vi "astrom_test.vi"() -> ()   [LabVIEW 2010]
panel:
  out "ImgRA [°]":dbl format="%.6f"
  out "ImgDEC [°]":dbl format="%.5f"
  in  "settablexy":bool
  in  "setpixel":bool
  in  "Image Y":dbl
  in  "Image X":dbl
  in  "RA":dbl format="%<%H:%M:%S%2u>t"
  in  "DEC":dbl format="%<%H:%M:%S%1u>t"
  out "ZoomIN":sgl[][](graph)
  in  "Table Y":dbl format="%.2f"
  in  "Table X":dbl format="%.2f"
  in  "setradec":bool
  in  "readcursor":bool
  out "Imgage Data":sgl[][](array[numeric])
  out "ImgRA [sec]":dbl format="%<%H:%M:%S%2u>t"
  out "ImgDEC [sec]":dbl format="%<%H:%M:%S%1u>t"
  in  "Plot Size [arcmin]":dbl
  in  "redraw":bool
  in  "extast":bool
  in  "quit":bool
  in  "DEC(DD:MM:SS)":dbl format="%<%H:%M:%S>t"
  in  "RA (HH:MM:SS.S)":dbl format="%<%H:%M:%S%1u>t"
  out "Field Astrometry":T1
  out "Table Astrometry":T1
  out "Image Astrometry":T1
  in  "Ref y (pas)":dbl
  in  "Ref x (pas)":dbl
  in  "effective rotation (°)":dbl step=5.0
  in  "scale (\"/pas)":dbl
  out "XY Graph":cluster{dbl[], dbl[]}[](graph)
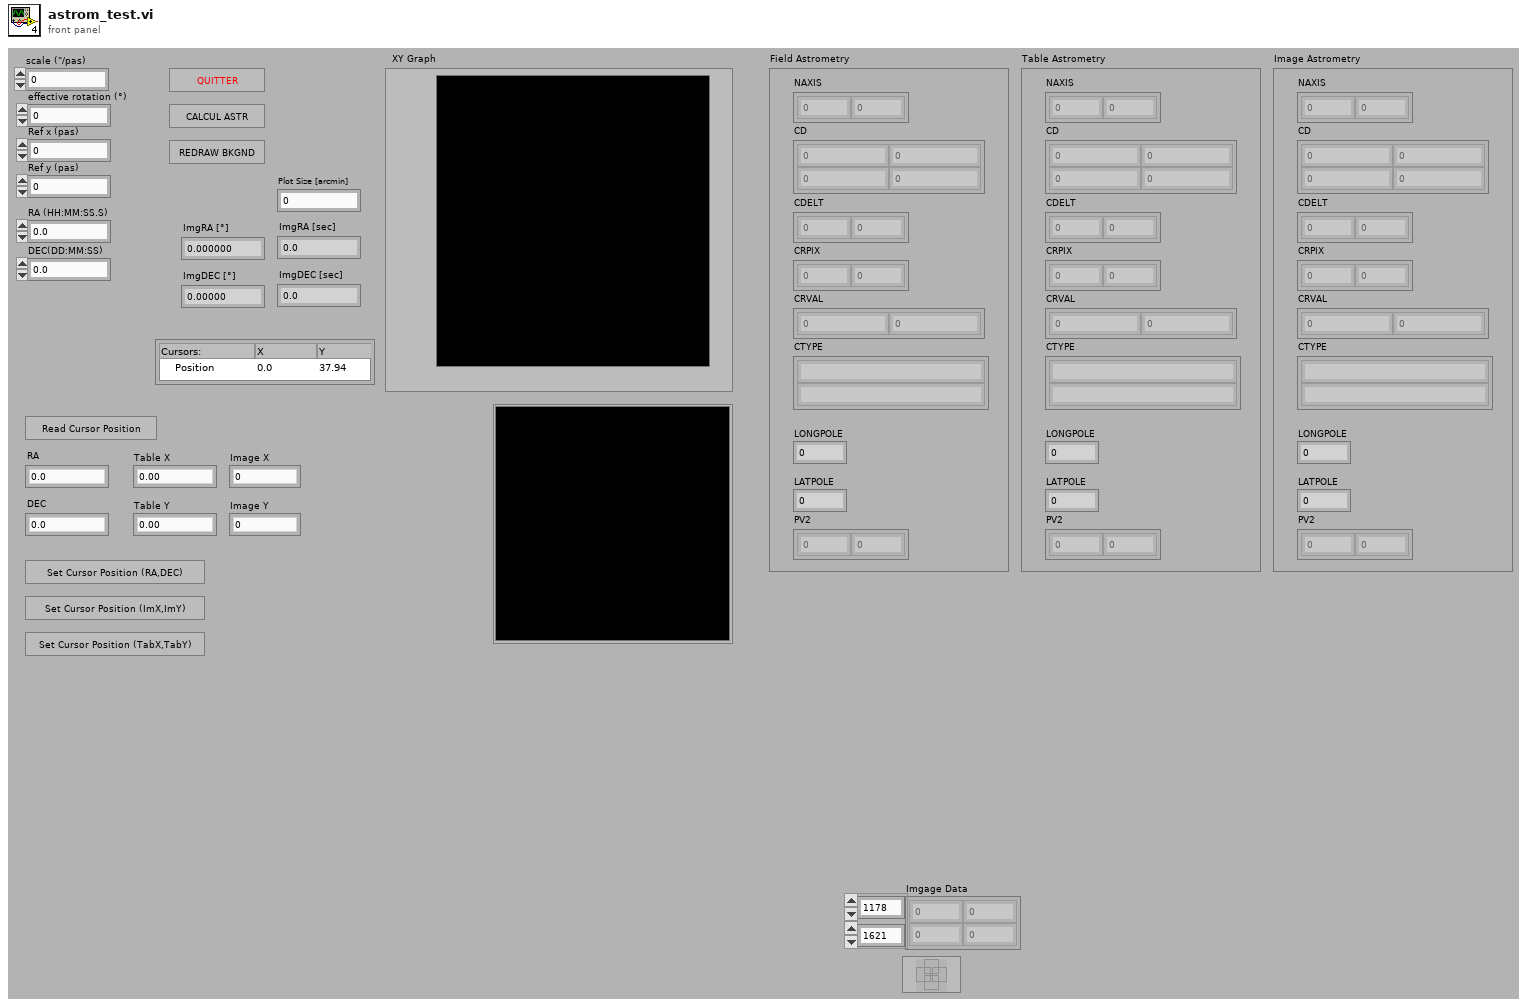
[diagram p1: front panel]
types:
  T1 = cluster{"NAXIS":dbl[], "CD":dbl[][], "CDELT":dbl[], "CRPIX":dbl[], "CTYPE":string[], "CRVAL":dbl[], "LONGPOLE":dbl, "LATPOLE":dbl, "PV2":dbl[]}
  T2 = typedef "LVRangeTypeDef.ctl" = cluster{"Minimum":dbl, "Maximum":dbl, "Increment":dbl, "Minor Increment":dbl, "Start":dbl}
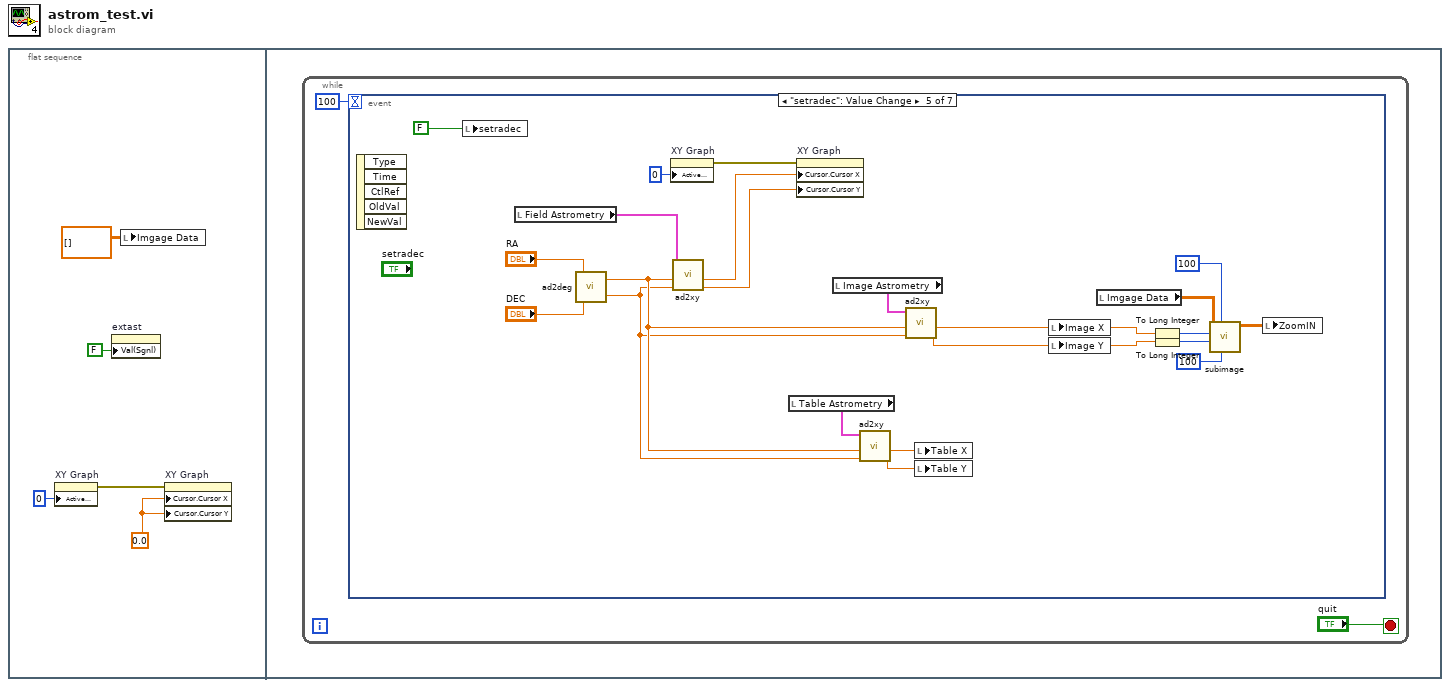
[diagram p0: block diagram]
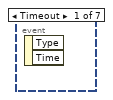
[diagram p2: hidden frame]
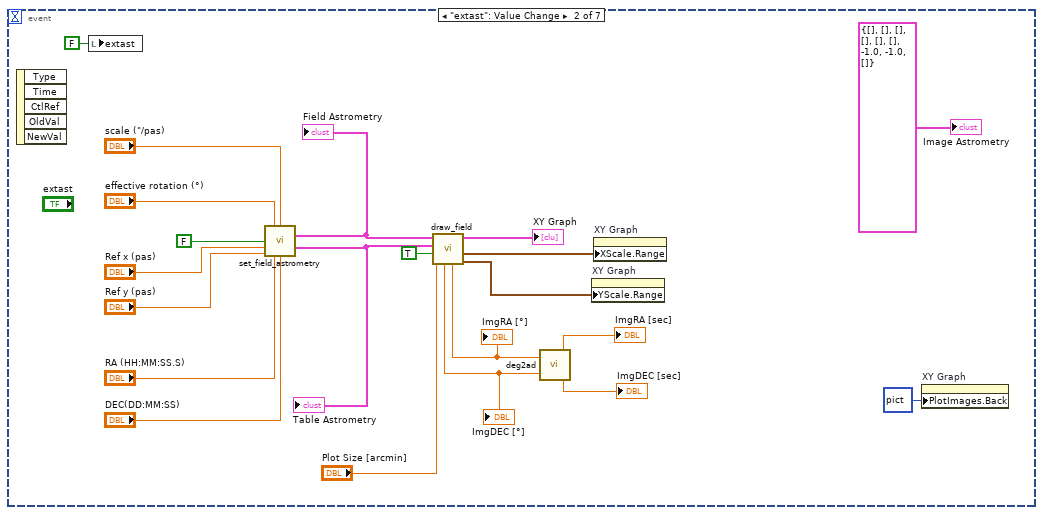
[diagram p3: hidden frame]
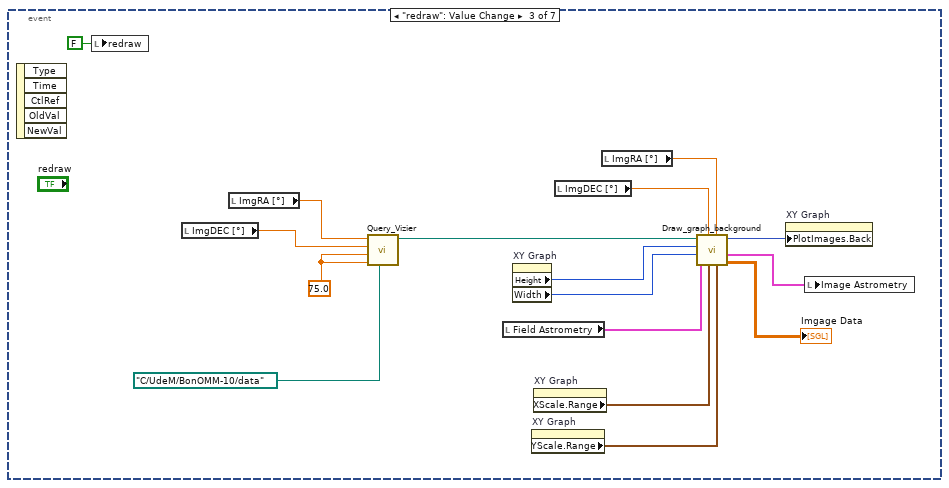
[diagram p4: hidden frame]
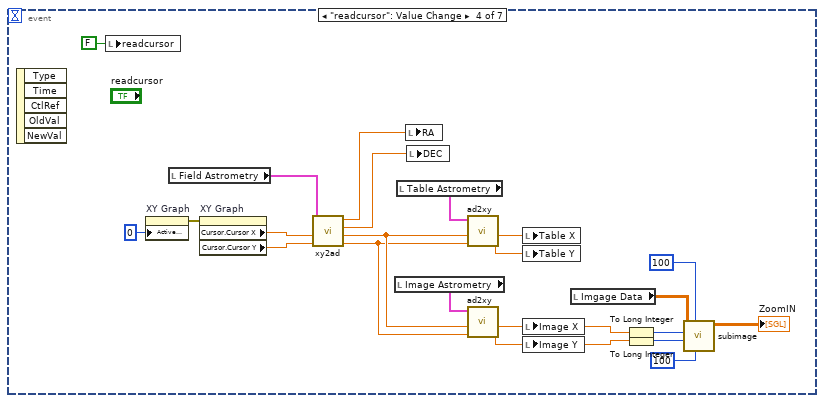
[diagram p5: hidden frame]
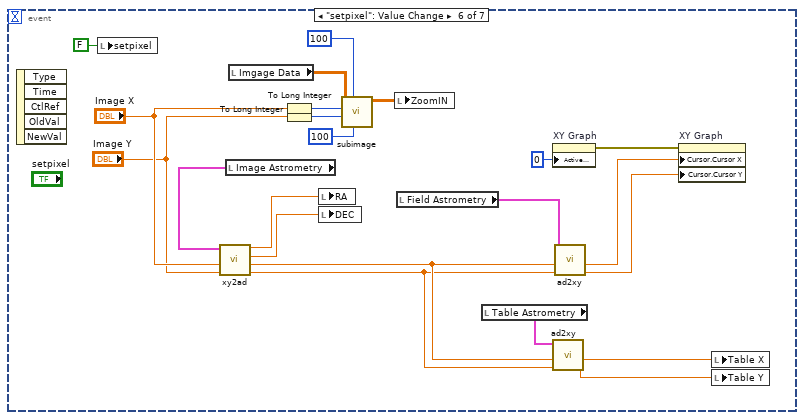
[diagram p6: hidden frame]
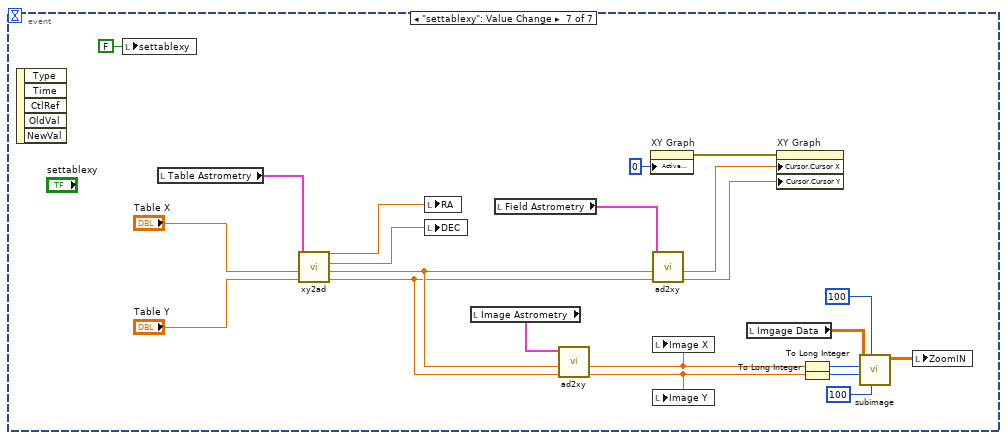
[diagram p7: hidden frame]
diagram:
  n1 = flat-sequence {
    frame #0 {
      w1 = 0.0
      n2 = property on="XY Graph" class="XYGraph (strict)"("Active Cursor"=u32 0) -> (error out=w2:errorcluster)  [unwired: 2 in, 1 out]
      n3 = property on="extast" class="Bool (strict)"("Val(Sgnl)"=FALSE ("Value (Signaling)")) -> ()  [unwired: 2 in, 2 out]
      n4 = local write "Imgage Data"(sgl[][] [] ("Imgage Data")) -> ()
      n5 = property on="XY Graph" class="XYGraph (strict)"(error in=w2, "Cursor.Cursor X"=w1, "Cursor.Cursor Y"=w1) -> ()  [unwired: 1 in, 2 out]
    }
    frame #1 {
      n6 = while {
        stop <- "quit" stop-if-true
        n7 = event shown="[4] \"setradec\": Value Change" {
          selector: _ -> [_ _ _ _ _ _ _]
          dyn-events: _ -> [_ _ _ _ _ _ _]
          timeout: 100 -> [_ _ _ _ _ _ _]
          event Timeout {
            n8 = event-data() -> ()  [unwired: 1 in, 2 out]
          }
          event "extast": Value Change {
            n9 = event-data() -> ()  [unwired: 1 in, 5 out]
            n10 = local write "extast"(FALSE ("extast")) -> ()
            n11 = call "set_field_astrometry.vi"("effective rotation (°)"="effective rotation (°)", "scale (\"/pas)"="scale (\"/pas)", "Use Center?"=FALSE, "Ref x (pas)"="Ref x (pas)", "Ref y (pas)"="Ref y (pas)", "RA (HH:MM:SS.S)"="RA (HH:MM:SS.S)", "DEC(DD:MM:SS)"="DEC(DD:MM:SS)") -> ("Field Astrometry"=w21:T1, "Table Astrometry"=w22:T1)  [unwired: 7 in]
            "Table Astrometry" <- w22
            "Field Astrometry" <- w21
            n12 = call "draw_field.vi"("margin/size"="Plot Size [arcmin]", "Ues Constant Size ?"=TRUE, "Table_Astrometry"=w22, "Field_Astrometry"=w21) -> ("Y Scale.Range"=w15:T2, "X Scale.Range"=w16:T2, "TableXYPos"=→"XY Graph":cluster{dbl[], dbl[]}[], "ImgRA"=w11:dbl, "ImgDEC"=w10:dbl)  [unwired: 3 in]
            "ImgRA [°]" <- w11
            "ImgDEC [°]" <- w10
            n13 = call "deg2ad.vi"("DEC (°)"=w10, "RA (°)"=w11) -> ("DEC (sec)"=→"ImgDEC [sec]":dbl, "RA (sec)"=→"ImgRA [sec]":dbl)
            n14 = property on="XY Graph" class="XYGraph (strict)"("YScale.Range"=w15) -> ()  [unwired: 2 in, 2 out]
            n15 = property on="XY Graph" class="XYGraph (strict)"("XScale.Range"=w16) -> ()  [unwired: 2 in, 2 out]
            n16 = property on="XY Graph" class="XYGraph (strict)"("PlotImages.Back"=picture data[5B] ("Plot Images:Back")) -> ()  [unwired: 2 in, 2 out]
            "Image Astrometry" <- T1 {"NAXIS"=[], "CD"=[], "CDELT"=[], "CRPIX"=[], "CTYPE"=[], "CRVAL"=[], "LONGPOLE"=-1.0, "LATPOLE"=-1.0, "PV2"=[]} ("Image Astrometry")
          }
          event "redraw": Value Change {
            w31 = 75.0 ("Height")
            n17 = event-data() -> ()  [unwired: 1 in, 5 out]
            n18 = local write "redraw"(FALSE ("redraw")) -> ()
            n19 = local read "ImgDEC [°]"() -> (w32:dbl)
            n20 = local read "ImgRA [°]"() -> (w33:dbl)
            n21 = call "Query_Vizier.vi"("Folder"=path "C:/UdeM/BonOMM-10/data", "Width"=w31, "Height"=w31, "DEC"=w32, "RA"=w33) -> ("Path2Image"=w29:path)  [unwired: 5 in, 1 out]
            n22 = local read "Field Astrometry"() -> (w40:T1)
            n23 = property on="XY Graph" class="XYGraph (strict)"() -> ("Height"=w42:u32, "Width"=w41:u32)  [unwired: 2 in, 2 out]
            n24 = property on="XY Graph" class="XYGraph (strict)"() -> ("YScale.Range"=w38:T2)  [unwired: 2 in, 2 out]
            n25 = property on="XY Graph" class="XYGraph (strict)"() -> ("XScale.Range"=w39:T2)  [unwired: 2 in, 2 out]
            n26 = local read "ImgDEC [°]"() -> (w36:dbl)
            n27 = local read "ImgRA [°]"() -> (w37:dbl)
            n28 = call "Draw_graph_background.vi"("Y Scale.Range"=w38, "ImgRA"=w37, "X Scale.Range"=w39, "ImgDEC"=w36, "Field Astrometry"=w40, "New Width"=w41, "New Height"=w42, "path"=w29) -> ("ImgData"=→"Imgage Data":sgl[][], "Astrometry"=w35:T1, "Images"=w43:picture)  [unwired: 1 in]
            n29 = property on="XY Graph" class="XYGraph (strict)"("PlotImages.Back"=w43) -> ()  [unwired: 2 in, 2 out]
            n30 = local write "Image Astrometry"(w35) -> ()
          }
          event "readcursor": Value Change {
            n31 = event-data() -> ()  [unwired: 1 in, 5 out]
            n32 = local write "readcursor"(FALSE ("readcursor")) -> ()
            n33 = property on="XY Graph" class="XYGraph (strict)"("Active Cursor"=u32 0) -> (error out=w65:errorcluster)  [unwired: 2 in, 1 out]
            n34 = local read "Field Astrometry"() -> (w62:T1)
            n35 = property on="XY Graph" class="XYGraph (strict)"(error in=w65) -> ("Cursor.Cursor X"=w64:dbl, "Cursor.Cursor Y"=w63:dbl)  [unwired: 1 in, 2 out]
            n36 = call "xy2ad.vi"("Y (px)"=w63, "X (px)"=w64, "Astrometry"=w62) -> ("DEC (°)"=w59:dbl, "RA (°)"=w60:dbl, "DEC (HH:MM:SS)"=w56:dbl, "RA (HH:MM:SS.S)"=w57:dbl)  [unwired: 5 in]
            n37 = local read "Image Astrometry"() -> (w58:T1)
            n38 = local read "Table Astrometry"() -> (w61:T1)
            n39 = local write "RA"(w57) -> ()
            n40 = local write "DEC"(w56) -> ()
            n41 = call "ad2xy.vi"("DEC"=w59, "RA"=w60, "Astrometry"=w61) -> ("Y"=w54:dbl, "X"=w55:dbl)  [unwired: 6 in, 1 out]
            n42 = call "ad2xy.vi"("DEC"=w59, "RA"=w60, "Astrometry"=w58) -> ("Y"=w50:dbl, "X"=w51:dbl)  [unwired: 6 in, 1 out]
            n43 = local write "Table X"(w55) -> ()
            n44 = local write "Table Y"(w54) -> ()
            n45 = local write "Image X"(w51) -> ()
            n46 = local write "Image Y"(w50) -> ()
            n47 = local read "Imgage Data"() -> (w47:sgl[][])
            n48 = To Long Integer(number=w51) -> (32bit integer=w53:i32)
            n49 = To Long Integer(number=w50) -> (32bit integer=w52:i32)
            n50 = call "subimage.vi"("Ysz/2"=100, "Xsz/2"=100, "Yc"=w52, "Xc"=w53, "ImgData"=w47) -> ("SubImg"=→"ZoomIN":sgl[][])  [unwired: 6 in]
          }
          event "setradec": Value Change {
            n51 = event-data() -> ()  [unwired: 1 in, 5 out]
            n52 = local write "setradec"(FALSE ("setcursor")) -> ()
            n53 = local read "Field Astrometry"() -> (w87:T1)
            n54 = call "ad2deg.vi"("DEC (sec)"="DEC", "RA (sec)"="RA") -> ("DEC (°)"=w67:dbl, "RA (°)"=w68:dbl)
            n55 = property on="XY Graph" class="XYGraph (strict)"("Active Cursor"=u32 0) -> (error out=w86:errorcluster)  [unwired: 2 in, 1 out]
            n56 = call "ad2xy.vi"("DEC"=w67, "RA"=w68, "Astrometry"=w87) -> ("Y"=w84:dbl, "X"=w85:dbl)  [unwired: 6 in, 1 out]
            n57 = local read "Table Astrometry"() -> (w74:T1)
            n58 = property on="XY Graph" class="XYGraph (strict)"(error in=w86, "Cursor.Cursor X"=w85, "Cursor.Cursor Y"=w84) -> ()  [unwired: 1 in, 2 out]
            n59 = local read "Image Astrometry"() -> (w82:T1)
            n60 = call "ad2xy.vi"("DEC"=w67, "RA"=w68, "Astrometry"=w74) -> ("Y"=w72:dbl, "X"=w73:dbl)  [unwired: 6 in, 1 out]
            n61 = call "ad2xy.vi"("DEC"=w67, "RA"=w68, "Astrometry"=w82) -> ("Y"=w78:dbl, "X"=w79:dbl)  [unwired: 6 in, 1 out]
            n62 = local write "Table X"(w73) -> ()
            n63 = local write "Table Y"(w72) -> ()
            n64 = local write "Image X"(w79) -> ()
            n65 = local write "Image Y"(w78) -> ()
            n66 = local read "Imgage Data"() -> (w75:sgl[][])
            n67 = To Long Integer(number=w79) -> (32bit integer=w81:i32)
            n68 = To Long Integer(number=w78) -> (32bit integer=w80:i32)
            n69 = call "subimage.vi"("Ysz/2"=100, "Xsz/2"=100, "Yc"=w80, "Xc"=w81, "ImgData"=w75) -> ("SubImg"=w83:sgl[][])  [unwired: 6 in]
            n70 = local write "ZoomIN"(w83) -> ()
          }
          event "setpixel": Value Change {
            n71 = event-data() -> ()  [unwired: 1 in, 5 out]
            n72 = local write "setpixel"(FALSE ("setpixel")) -> ()
            n73 = local read "Image Astrometry"() -> (w101:T1)
            n74 = call "xy2ad.vi"("Y (px)"="Image Y", "X (px)"="Image X", "Astrometry"=w101) -> ("DEC (°)"=w90:dbl, "RA (°)"=w91:dbl, "DEC (HH:MM:SS)"=w99:dbl, "RA (HH:MM:SS.S)"=w100:dbl)  [unwired: 5 in]
            n75 = local read "Imgage Data"() -> (w104:sgl[][])
            n76 = To Long Integer(number="Image X") -> (32bit integer=w108:i32)
            n77 = To Long Integer(number="Image Y") -> (32bit integer=w107:i32)
            n78 = local write "RA"(w100) -> ()
            n79 = local write "DEC"(w99) -> ()
            n80 = call "subimage.vi"("Ysz/2"=100, "Xsz/2"=100, "Yc"=w107, "Xc"=w108, "ImgData"=w104) -> ("SubImg"=w109:sgl[][])  [unwired: 6 in]
            n81 = local write "ZoomIN"(w109) -> ()
            n82 = local read "Field Astrometry"() -> (w98:T1)
            n83 = local read "Table Astrometry"() -> (w94:T1)
            n84 = property on="XY Graph" class="XYGraph (strict)"("Active Cursor"=u32 0) -> (error out=w97:errorcluster)  [unwired: 2 in, 1 out]
            n85 = call "ad2xy.vi"("DEC"=w90, "RA"=w91, "Astrometry"=w94) -> ("Y"=w92:dbl, "X"=w93:dbl)  [unwired: 6 in, 1 out]
            n86 = call "ad2xy.vi"("DEC"=w90, "RA"=w91, "Astrometry"=w98) -> ("Y"=w95:dbl, "X"=w96:dbl)  [unwired: 6 in, 1 out]
            n87 = property on="XY Graph" class="XYGraph (strict)"(error in=w97, "Cursor.Cursor X"=w96, "Cursor.Cursor Y"=w95) -> ()  [unwired: 1 in, 2 out]
            n88 = local write "Table X"(w93) -> ()
            n89 = local write "Table Y"(w92) -> ()
          }
          event "settablexy": Value Change {
            n90 = event-data() -> ()  [unwired: 1 in, 5 out]
            n91 = local write "settablexy"(FALSE ("settablexy")) -> ()
            n92 = local read "Table Astrometry"() -> (w129:T1)
            n93 = call "xy2ad.vi"("Y (px)"="Table Y", "X (px)"="Table X", "Astrometry"=w129) -> ("DEC (°)"=w119:dbl, "RA (°)"=w120:dbl, "DEC (HH:MM:SS)"=w127:dbl, "RA (HH:MM:SS.S)"=w128:dbl)  [unwired: 5 in]
            n94 = local write "RA"(w128) -> ()
            n95 = local write "DEC"(w127) -> ()
            n96 = local read "Image Astrometry"() -> (w121:T1)
            n97 = local read "Field Astrometry"() -> (w126:T1)
            n98 = call "ad2xy.vi"("DEC"=w119, "RA"=w120, "Astrometry"=w121) -> ("Y"=w111:dbl, "X"=w112:dbl)  [unwired: 6 in, 1 out]
            n99 = property on="XY Graph" class="XYGraph (strict)"("Active Cursor"=u32 0) -> (error out=w125:errorcluster)  [unwired: 2 in, 1 out]
            n100 = call "ad2xy.vi"("DEC"=w119, "RA"=w120, "Astrometry"=w126) -> ("Y"=w123:dbl, "X"=w124:dbl)  [unwired: 6 in, 1 out]
            n101 = local write "Image X"(w112) -> ()
            n102 = local write "Image Y"(w111) -> ()
            n103 = local read "Imgage Data"() -> (w113:sgl[][])
            n104 = property on="XY Graph" class="XYGraph (strict)"(error in=w125, "Cursor.Cursor X"=w124, "Cursor.Cursor Y"=w123) -> ()  [unwired: 1 in, 2 out]
            n105 = To Long Integer(number=w112) -> (32bit integer=w117:i32)
            n106 = To Long Integer(number=w111) -> (32bit integer=w116:i32)
            n107 = call "subimage.vi"("Ysz/2"=100, "Xsz/2"=100, "Yc"=w116, "Xc"=w117, "ImgData"=w113) -> ("SubImg"=w118:sgl[][])  [unwired: 6 in]
            n108 = local write "ZoomIN"(w118) -> ()
          }
        }
      }
    }
  }
